vi "FichierTest.vi"() -> ()   [LabVIEW 2020]
uses:
  <vilib>/Utility/xml.llb/Write to XML File(string).vi
panel:
  out "XML String":string
  in  "ID 2":cluster{"Nom":string, "Age":u8, "Prenom":string}
  out "data":cluster{"Nom":string, "Age":u8, "Prenom":string}
  in  "ID":cluster{"Nom":string, "Age":u8, "Prenom":string}
  out "text":string
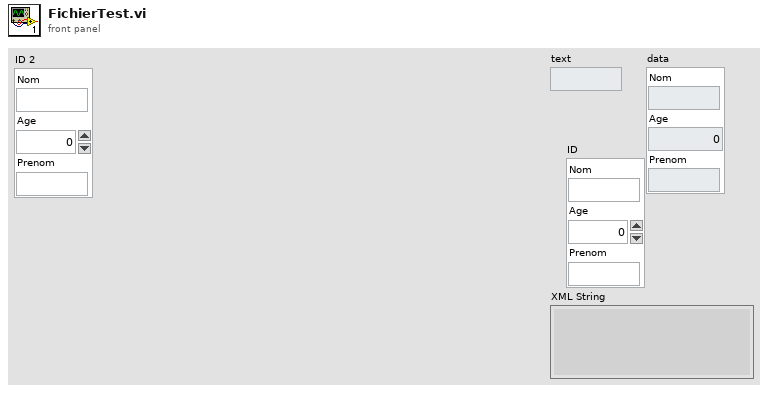
[diagram p1: front panel]
types:
  T1 = enum16{"big-endian, network order", "native, host order", "little-endian"}
  T2 = enum16{"open", "replace", "create", "open or create", "replace or create", "replace or create with confirmation"}
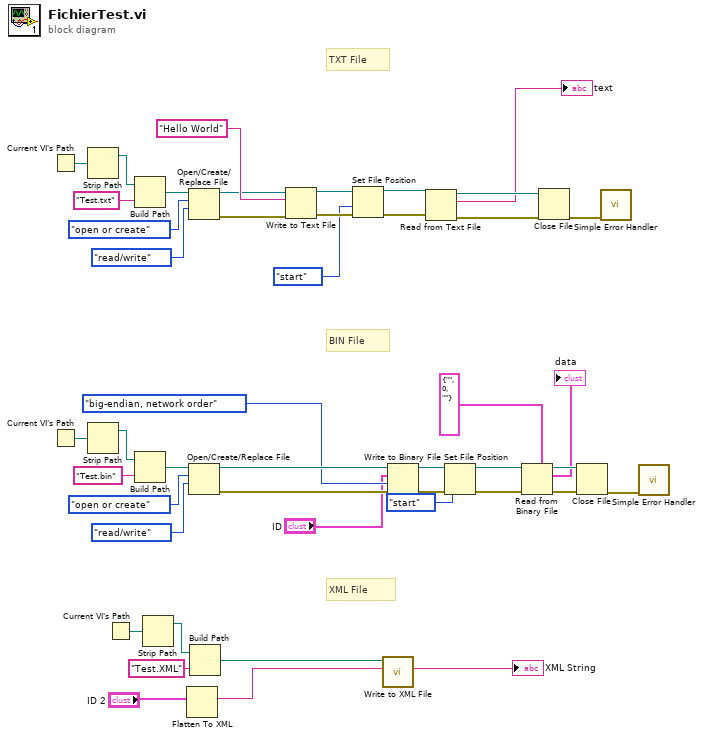
[diagram p0: block diagram]
diagram:
  # "XML File"
  # "BIN File"
  # "TXT File"
  n1 = Current VI's Path() -> (path=w45:path)
  n2 = Current VI's Path() -> (path=w23:path)
  n3 = Strip Path(path=w45) -> (stripped path=w35:path)  [unwired: 1 out]
  n4 = Strip Path(path=w23) -> (stripped path=w27:path)  [unwired: 1 out]
  n5 = Current VI's Path() -> (path=w7:path)
  n6 = Build Path(base path=w35, name or relative path="Test.txt") -> (appended path=w33:path)
  n7 = Build Path(base path=w27, name or relative path="Test.bin") -> (appended path=w28:path)
  n8 = Strip Path(path=w7) -> (stripped path=w5:path)  [unwired: 1 out]
  n9 = Flatten To XML(6:"ID 2") -> (2:w2:string)
  n10 = Open/Create/Replace File(file path (use dialog)=w33, operation (0:open)=T2."open or create", access (0:read/write)=enum16{"read/write", "read-only", "write-only"}."read/write") -> (refnum out=w34:refnum<file>, error out=w38:errorcluster)  [unwired: 3 in, 1 out]
  n11 = Open/Create/Replace File(file path (use dialog)=w28, operation (0:open)=T2."open or create", access (0:read/write)=enum16{"read/write", "read-only", "write-only"}."read/write") -> (refnum out=w22:refnum<file>, error out=w20:errorcluster)  [unwired: 3 in, 1 out]
  n12 = Build Path(base path=w5, name or relative path="Test.XML") -> (appended path=w4:path)
  n13 = Write to Text File(file (use dialog)=w34, text="Hello World", error in=w38) -> (refnum out=w31:refnum<file>, error out=w32:errorcluster)  [unwired: 1 in, 1 out]
  n14 = Set File Position(refnum=w31, from (0:start)=enum16{"start", "end", "current"}."start", error in=w32) -> (refnum out=w29:refnum<file>, error out=w30:errorcluster)  [unwired: 1 in]
  n15 = call-poly <vilib>:"Write to XML File.vi"("XML Input"=w2, "XML File Path"=w4) -> ("XML String"=→"XML String":string)  [unwired: 7 in, 2 out]
  n16 = Write to Binary File(file (use dialog)=w22, data="ID", error in=w20, 9:T1."big-endian, network order" ("byte order (0:big-endian, network order)")) -> (refnum out=w17:refnum<file>, error out=w18:errorcluster)  [unwired: 2 in, 1 out]
  n17 = Read from Text File(file (use dialog)=w29, error in=w30) -> (refnum out=w41:refnum<file>, text=→"text":string, error out=w40:errorcluster)  [unwired: 2 in, 1 out]
  n18 = Set File Position(refnum=w17, from (0:start)=enum16{"start", "end", "current"}."start", error in=w18) -> (refnum out=w14:refnum<file>, error out=w15:errorcluster)  [unwired: 1 in]
  n19 = Read from Binary File(5:cluster{"Nom":string, "Age":u8, "Prenom":string} {"Nom"="", "Age"=0, "Prenom"=""} ("ID 2"), 8:w15, 11:w14) -> (0:w12:errorcluster, 2:→"data":cluster{"Nom":string, "Age":u8, "Prenom":string}, 3:w11:refnum<file>)  [unwired: 3 in, 1 out]
  n20 = Close File(refnum=w41, error in=w40) -> (error out=w36:errorcluster)  [unwired: 1 out]
  n21 = Close File(refnum=w11, error in=w12) -> (error out=w13:errorcluster)  [unwired: 1 out]
  n22 = call <vilib>:"Simple Error Handler.vi"("error in (no error)"=w36) -> ()  [unwired: 4 in, 5 out]
  n23 = call <vilib>:"Simple Error Handler.vi"("error in (no error)"=w13) -> ()  [unwired: 4 in, 5 out]
